vi "Scan Time (str) (SubVI).vi"(6 "字符串":string, 9 "queue out输入":refnum<queue>, 11 "队列输入":refnum<queue>) -> (0 "错误输出":errorcluster)   [LabVIEW 2019, in "Take Seq.lvlib"]
uses:
  Take Seq.lvlib
  error.ctl
  lib/QDInstrument.dll
  SubVI.lvlib
panel:
  # "(真是通道1，假是通道2)"
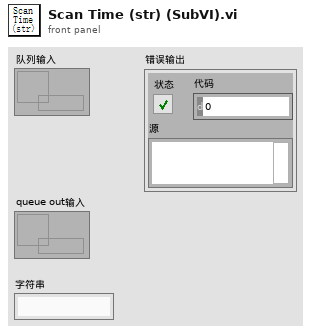
[diagram p1: front panel]
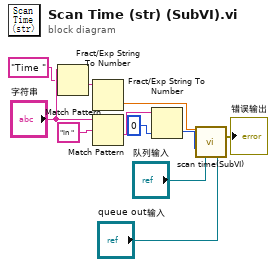
[diagram p0: block diagram]
diagram:
  n1 = Match Pattern(string="字符串", regular expression="Time " ("正则表达式")) -> (after substring=w4:string)  [unwired: 1 in, 3 out]
  n2 = Fract/Exp String To Number(string=w4) -> (number=w5:dbl)  [unwired: 3 in, 1 out]
  n3 = Match Pattern(string="字符串", regular expression="in " ("正则表达式")) -> (after substring=w9:string)  [unwired: 1 in, 3 out]
  n4 = Fract/Exp String To Number(string=w9, default (0 dbl)=0) -> (number=w6:i32)  [unwired: 2 in, 1 out]
  n5 = call "scan time(SubVI).vi"("total time"=w5, "steps number"=w6, "data"="队列输入", "config"="queue out输入") -> ("错误输出"=→"错误输出":errorcluster)  [unwired: 11 in]
